vi "Launch Compass Actor.vi"(7 "Sim?":bool, 11 "RDS Root Actor in":refnum<class "RDS Root Actor.lvclass">) -> (3 "RDS Root Actor out":refnum<class "RDS Root Actor.lvclass">)   [LabVIEW 2015, in "RDS Root Actor.lvlib" / "RDS Root Actor.lvclass"]
uses:
  RDS Root Actor.lvclass
  Libraries/RDS Framework/RDS Message ID.ctl
  Libraries/RDS Instruments/Compass Instrument/Compass Instrument.lvclass
  Libraries/RDS Instruments/RDS Instrument Enums.ctl
  Libraries/RDS Instruments/Compass Instrument/Compass Instrument.lvclass/Compass Instrument.ctl
  RDS Parent Actor/RDS Parent Actor/RDS Parent Actor.lvclass/RDS Parent Actor.ctl
  RDS Serial Instrument Actor/RDS Serial Instrument Actor.lvclass/RDS Serial Instrument Actor.ctl
  Sim/Sim Compass/Sim Compass/Sim Compass/Sim Compass.lvclass
  RDS Parent Actor/RDS Parent Actor/RDS Parent Actor.lvclass
  RDS Serial Instrument Actor/RDS Serial Instrument Actor.lvclass
  Libraries/RDS Child Messages/RDS Child Messages.lvlib
  Libraries/Configuration Library/RDS Configuration Library.lvlib
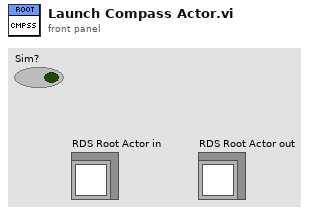
[diagram p1: front panel]
types:
  T1 = typedef "RDS Configuration Library.lvlib/RDS Instrument Enums.ctl" = enum16{"AIP", "GPS", "Compass", "PORT Motor", "STBD Motor", "LSR", "Depth Transducer", "BTB"}
  T2 = typedef "RDS Child Messages.lvlib/RDS Message ID.ctl" = enum16{"RDS Hello World", "String Message", "AIP_Status", "AIP_Command", "GPS_Data", "MCB_Command", "MCB_Status", "Compass_Data", "Depth_Data", "Battery_Data", "Contoller_State", "Set_Mag_Dev", "BTB_Shutdown", "State_Sample_Request", "State_Sample", "PID_Gains_Set", "Helm_Limiter_Set", "Helm_Heading_Command", "Helm_Steering_Command", "Helm_Status", "Controller_Message", "AIP_Set_Min_Depth", "Mission_Controller_State", "Mission_Upload", "Mission_Set_Op_and_Run", "Mission_Settings_Set"}
  T3 = typedef "RDS Configuration Library.lvlib/RDS Configuration.ctl" = cluster{"State Update Rate (Hz)":dbl, "Helm Rate (Hz)":dbl, "Helm Gains":T4, "Limiter":dbl, "Mission Controller Settings":T5, "Mag Dev":dbl}
  T4 = typedef "RDS Child Messages.lvlib/PID Gains Control.ctl" = cluster{"P (Kc)":sgl, "I (Ti)":sgl, "D (Td)":sgl}
  T5 = typedef "RDS Mission Controller Actor.lvlib/Mission Controller Settings.ctl" = cluster{"Waypoint Radius (m)":dbl}
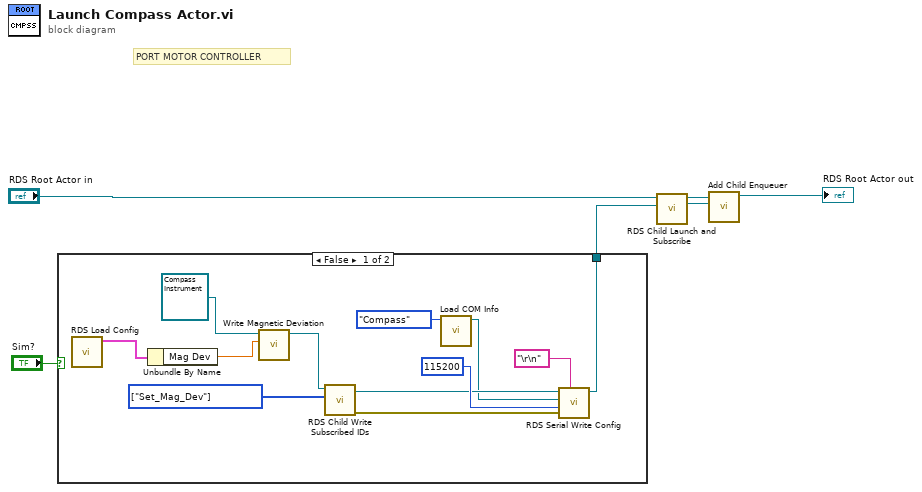
[diagram p0: block diagram]
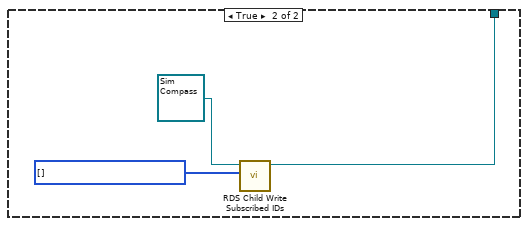
[diagram p2: hidden frame]
diagram:
  # "PORT MOTOR CONTROLLER"
  n1 = case shown="False" "Sim?" {
    tunnel: [w18 w19] -> w2
    frame False {
      w15 = T2[] [enum."Set_Mag_Dev"] items=["RDS Hello World", "String Message", "AIP_Status", "AIP_Command", "GPS_Data", "MCB_Command", "MCB_Status", "Compass_Data", "Depth_Data", "Battery_Data", "Contoller_State", "Set_Mag_Dev", "BTB_Shutdown", "State_Sample_Request", "State_Sample", "PID_Gains_Set", "Helm_Limiter_Set", "Helm_Heading_Command", "Helm_Steering_Command", "Helm_Status", "Controller_Message", "AIP_Set_Min_Depth", "Mission_Controller_State", "Mission_Upload", "Mission_Set_Op_and_Run", "Mission_Settings_Set"] ("Subscribed IDs")
      n2 = call "RDS Load Config.vi"() -> ("RDS Config"=w10:T3)  [unwired: 11 in]
      n3 = Unbundle By Name(w10) -> ("Mag Dev"=w7:dbl)
      n4 = call "Write Magnetic Deviation.vi"("Magnetic Deviation"=w7, "Compass Instrument in"=refnum<class "Compass Instrument.lvclass"> refnum ("Compass Instrument.lvlib:Compass Instrument.lvclass")) -> ("Compass Instrument out"=w8:refnum<class "Compass Instrument.lvclass">)  [unwired: 8 in, 1 out]
      n5 = call "RDS Child Write Subscribed IDs.vi"("Subscribed IDs"=w15, "RDS Parent Actor in"=w8) -> ("error out"=w14:errorcluster, "RDS Parent Actor out"=w13:refnum<class "Compass Instrument.lvclass">)  [unwired: 8 in]
      n6 = call "Load COM Info.vi"("Serial Instrument"=RDS_Instrument_Enums."Compass") -> ("COM Port"=w11:refnum<visa-resource-name>)  [unwired: 10 in]
      n7 = call "RDS Serial Write Config.vi"("Termination Char(s)"="\r\n", "error in (no error)"=w14, "baud rate"=u32 115200, "VISA resource name"=w11, "RDS Serial Instrument Actor in"=w13) -> ("RDS Serial Instrument Actor out"=w18:refnum<class "Compass Instrument.lvclass">)  [unwired: 5 in, 1 out]
    }
    frame True {
      w21 = T2[] [] items=["RDS Hello World", "String Message", "AIP_Status", "AIP_Command", "GPS_Data", "MCB_Command", "MCB_Status", "Compass_Data", "Depth_Data", "Battery_Data", "Contoller_State", "Set_Mag_Dev", "BTB_Shutdown", "State_Sample_Request", "State_Sample", "PID_Gains_Set", "Helm_Limiter_Set", "Helm_Heading_Command", "Helm_Steering_Command", "Helm_Status", "Controller_Message", "AIP_Set_Min_Depth", "Mission_Controller_State", "Mission_Upload", "Mission_Set_Op_and_Run", "Mission_Settings_Set"] ("Subscribed IDs")
      n8 = call "RDS Child Write Subscribed IDs.vi"("Subscribed IDs"=w21, "RDS Parent Actor in"=refnum<class "Sim Compass.lvclass"> refnum ("Sim Compass.lvlib:Sim Compass.lvclass")) -> ("RDS Parent Actor out"=w19:refnum<class "Sim Compass.lvclass">)  [unwired: 8 in, 1 out]
    }
  }
  n9 = call "RDS Child Launch and Subscribe.vi"("RDS Child in"=w2, "Caller Actor in"="RDS Root Actor in") -> ("Nested Actor's Enqueuer"=w5:refnum<class "Message Enqueuer.lvclass">, "Caller Actor Out"=w4:refnum<class "RDS Root Actor.lvclass">)  [unwired: 7 in, 1 out]
  n10 = call "Add Child Enqueuer.vi"("Nested Actor's Enqueuer"=w5, "RDS Root Actor in"=w4) -> ("RDS Root Actor out"=→"RDS Root Actor out":refnum<class "RDS Root Actor.lvclass">)  [unwired: 8 in, 1 out]
